vi "Stop Robot Button.vi"() -> ()   [LabVIEW 2015]
panel:
  in  "?":bool
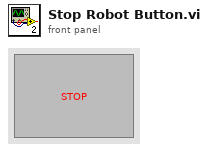
[diagram p1: front panel]
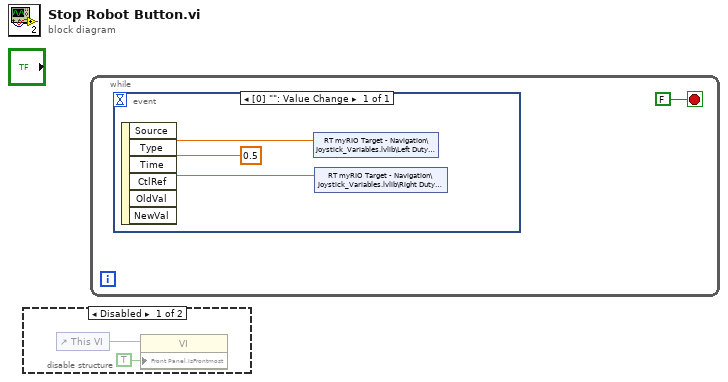
[diagram p0: block diagram]
diagram:
  n1 = disable-structure shown="Disabled" {
    frame Disabled {
      n2 = control-ref of="This VI"() -> (w2:refnum<vi>)
      n3 = property class="VI"(reference=w2, "Front Panel.IsFrontmost"=TRUE ("Front Panel Window:Is Frontmost")) -> ()  [unwired: 1 in, 2 out]
    }
    frame Enabled {
    }
  }
  n4 = while {
    stop <- FALSE stop-if-true
    n5 = event shown="[0] \"\": Value Change" {
      selector: _ -> [_]
      dyn-events: _ -> [_]
      timeout: _ -> [_]
      event Value Change {
        w4 = 0.5
        n6 = event-data() -> ()  [unwired: 1 in, 6 out]
        n7 = shared-variable "RT myRIO Target - Navigation\\Joystick_Variables.lvlib\\Left Duty Cycle"(w4) -> ()  [unwired: 1 in, 1 out]
        n8 = shared-variable "RT myRIO Target - Navigation\\Joystick_Variables.lvlib\\Right Duty Cycle"(w4) -> ()  [unwired: 1 in, 1 out]
      }
    }
  }
